vi "Streamline0002.vi"   [LabVIEW 2013]
uses:
  <vilib>/Heliosphere Research LLC/Advanced Plotting Toolkit/Advanced Plotting Toolkit.lvlib
types:
  T1 = typedef "Advanced Plotting Toolkit.lvlib/PlotID.ctl" = i32
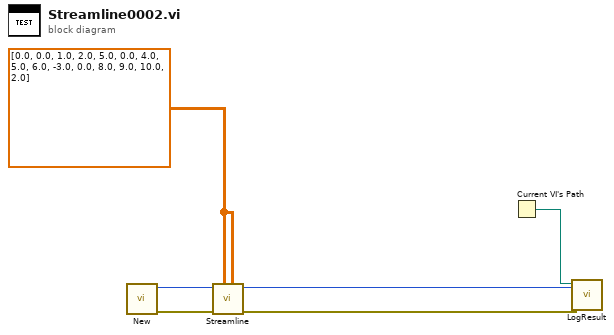
[diagram p0: block diagram]
diagram:
  w5 = dbl[][] [[0.0, 0.0, 1.0, 2.0, 5.0], [0.0, 4.0, 5.0, 6.0, -3.0], [0.0, 8.0, 9.0, 10.0, 2.0]] ("Data")
  n1 = call <vilib>:"New.vi"() -> ("error out"=w3:errorcluster, "Plot ID"=w4:T1)  [unwired: 10 in]
  n2 = call <vilib>:"Streamline.vi"("Y Vector Component"=w5, "X Vector Component"=w5, "error in (no error)"=w3, "Plot ID"=w4) -> ("error out"=w1:errorcluster, "Plot ID Out"=w2:T1)  [unwired: 6 in]
  n3 = Current VI's Path() -> (path=w6:path)
  n4 = call "LogResult.vi"("Test Result"=w1, "Test Artifact"=w2, "VI Path"=w6) -> ()  [unwired: 9 in]
